vi "Get Output Ref.vi"(8 "error in (no error)":errorcluster, 11 "output_request_poller in":refnum<class "output_poller.lvclass">) -> (0 "error out":errorcluster, 2 "output_ref":refnum<data-value>, 3 "output_request_poller out":refnum<class "output_poller.lvclass">)   [LabVIEW 2015, in "output_poller.lvclass"]
uses:
  output_poller.lvclass
  Output.lvclass
  output_poller.lvclass/output_poller.ctl
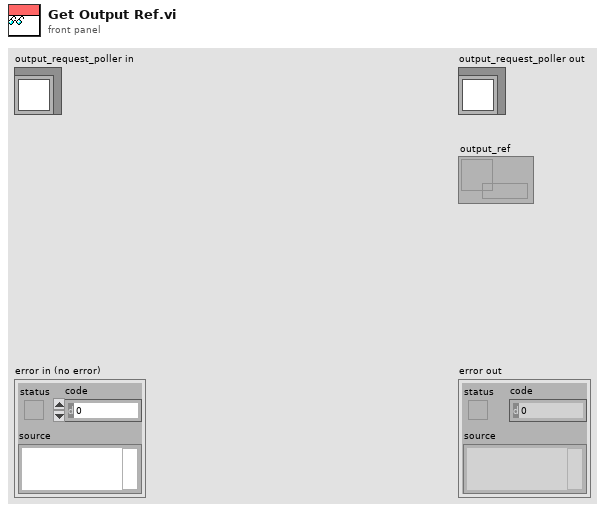
[diagram p1: front panel]
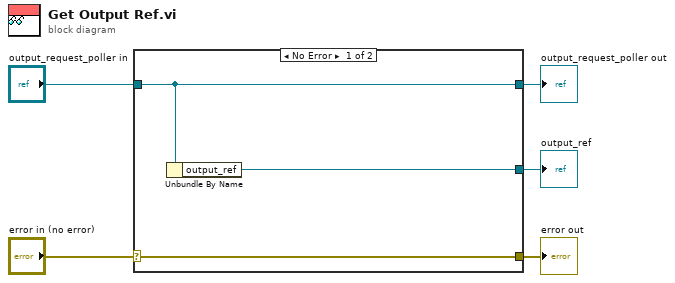
[diagram p0: block diagram]
diagram:
  n1 = case shown="No Error" "error in (no error)" {
    selector: "error in (no error)" -> [w8 w9]
    tunnel: [w8 w9] -> w4
    tunnel: [w7 w10] -> w2
    tunnel: "output_request_poller in" -> [w7 w10]
    tunnel: [w6 _] -> w1
    frame No Error {
      n2 = Unbundle By Name(w7) -> ("output_ref"=w6:refnum<data-value>)
    }
    frame Error {
    }
  }
  "error out" <- w4
  "output_request_poller out" <- w2
  "output_ref" <- w1
